vi "init.vi"(8 "error in (no error)":errorcluster, 11 "Stresing_dual_cam in":refnum<class "Stresing_dual_cam.lvclass">) -> (0 "error out":errorcluster, 3 "Stresing_dual_cam out":refnum<class "Stresing_dual_cam.lvclass">)   [LabVIEW 2019, in "Stresing_dual_cam.lvclass"]
uses:
  Stresing_dual_cam.lvclass
  Stresing_dual_cam.lvclass/Stresing_dual_cam.ctl
  _cameraBase/_cameraBase.lvclass
panel:
  out "wait time":dbl
  in  "nob":u32=1
  in  "nos":u32=1010
  in  "exposure":dbl=0.001
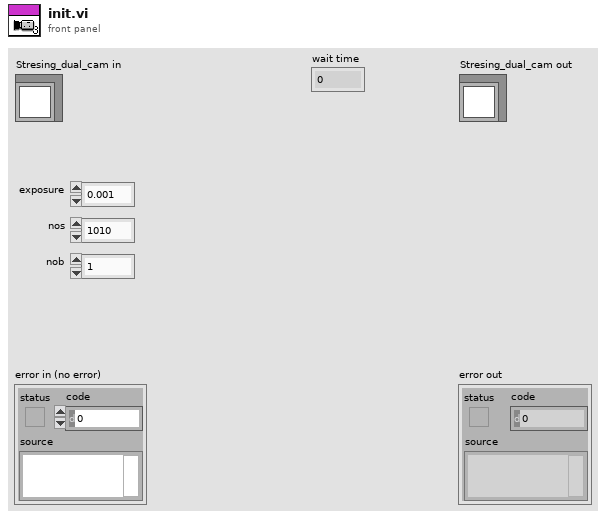
[diagram p1: front panel]
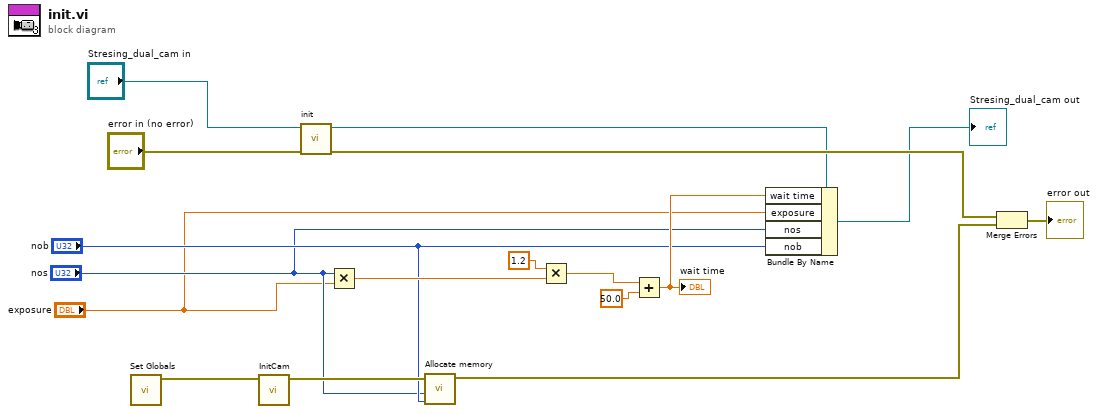
[diagram p0: block diagram]
diagram:
  n1 = call <instrlib>:"Set Globals.vi"() -> ("Camera error out"=w15:errorcluster)  [unwired: 11 in]
  n2 = call <instrlib>:"InitCam.vi"("Camera error in"=w15) -> ("Camera error out"=w14:errorcluster)  [unwired: 10 in]
  n3 = call-parent "init.vi"("error in (no error)"="error in (no error)", "_cameraBase in"="Stresing_dual_cam in") -> ("error out"=w9:errorcluster, "_cameraBase out"=w6:refnum<class "Stresing_dual_cam.lvclass">)  [unwired: 8 in]
  n4 = Multiply(x="nos", y="exposure") -> (x*y=w13:dbl)
  n5 = call <instrlib>:"Allocate memory.vi"("nob"="nob", "nos"="nos", "Camera error in"=w14) -> ("Camera error out"=w7:errorcluster)  [unwired: 8 in]
  n6 = Multiply(x=1.2, y=w13) -> (x*y=w11:dbl)
  n7 = Add(x=w11, y=50.0) -> (x+y=w4:dbl)
  "wait time" <- w4
  n8 = Bundle By Name(cluster=w6, "wait time"=w4, "exposure"="exposure", "nos"="nos", "nob"="nob") -> (→"Stresing_dual_cam out":refnum<class "Stresing_dual_cam.lvclass">)
  n9 = Merge Errors(w9, w7) -> (→"error out":errorcluster)
